vi "Required Locks.vi"(1 "Valves Per Reactor":i32=7, 4 "Valves":i32[](array[numeric])) -> (0 "Required Locks":i32[](array[numeric]))   [LabVIEW 2020]
doc: "Given a list of valves (1-40), converts to an array of required locks (0-2 or 3-inf)"
panel:
  out "x-y*floor(x/y)":i32
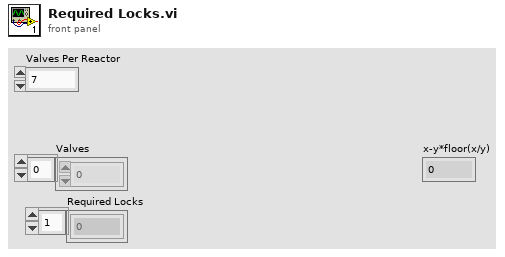
[diagram p1: front panel]
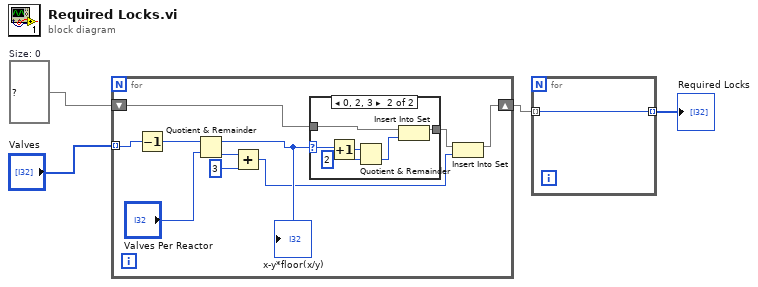
[diagram p0: block diagram]
diagram:
  w3 = set{i32} {}  # Size: 0
  n1 = for {
    tunnel: "Valves" -> [w14] mode=indexing
    shift-right: [w5] -> w2
    shift-left: w3 -> [w8]
    n2 = Decrement(x=w14) -> (x-1=w12:i32)
    n3 = Quotient & Remainder(x=w12, y="Valves Per Reactor") -> (x-y*floor(x/y)=w9:i32, floor(x/y)=w11:i32)
    "x-y*floor(x/y)" <- w9
    n4 = Add(x=w11, y=3) -> (x+y=w6:i32)
    n5 = case shown="0, 2, 3" w9 {
      selector: w9 -> [_ w20]
      tunnel: w8 -> [w15 w21]
      tunnel: [w15 w16] -> w7
      frame Default {
      }
      frame 0, 2, 3 {
        n6 = Increment(x=w20) -> (x+1=w19:i32)
        n7 = Quotient & Remainder(x=w19, y=2) -> (floor(x/y)=w17:i32)  [unwired: 1 out]
        n8 = Insert Into Set(10:w17, 11:w21) -> (3:w16:set{i32})  [unwired: 1 out]
      }
    }
    n9 = Insert Into Set(10:w6, 11:w7) -> (3:w5:set{i32})  [unwired: 1 out]
  }
  n10 = for {
    tunnel: [w22] -> w1 mode=indexing
    tunnel: w2 -> [w22] mode=indexing
  }
  "Required Locks" <- w1
